vi "CLD 10 Step Sequencer with CSV Front Panel.vi"() -> ()   [LabVIEW 2025]
doc: "CLD 10 Exercise"
uses:
  CLD 10 CSV file enum.ctl
panel:
  out "Elapsed Time (s)":string
  in  "Auto Reset":bool=TRUE
  in  "Reset Button":bool
  in  "Stop VI":bool
  in  "Time Target (s)":dbl
  out "Current Step Time":dbl
  out "Step 1":bool
  out "Step 2":bool
  out "Step 3":bool
  out "Time Has Elapsed":bool
  out "error out":errorcluster
  in  "error in (no error)":errorcluster
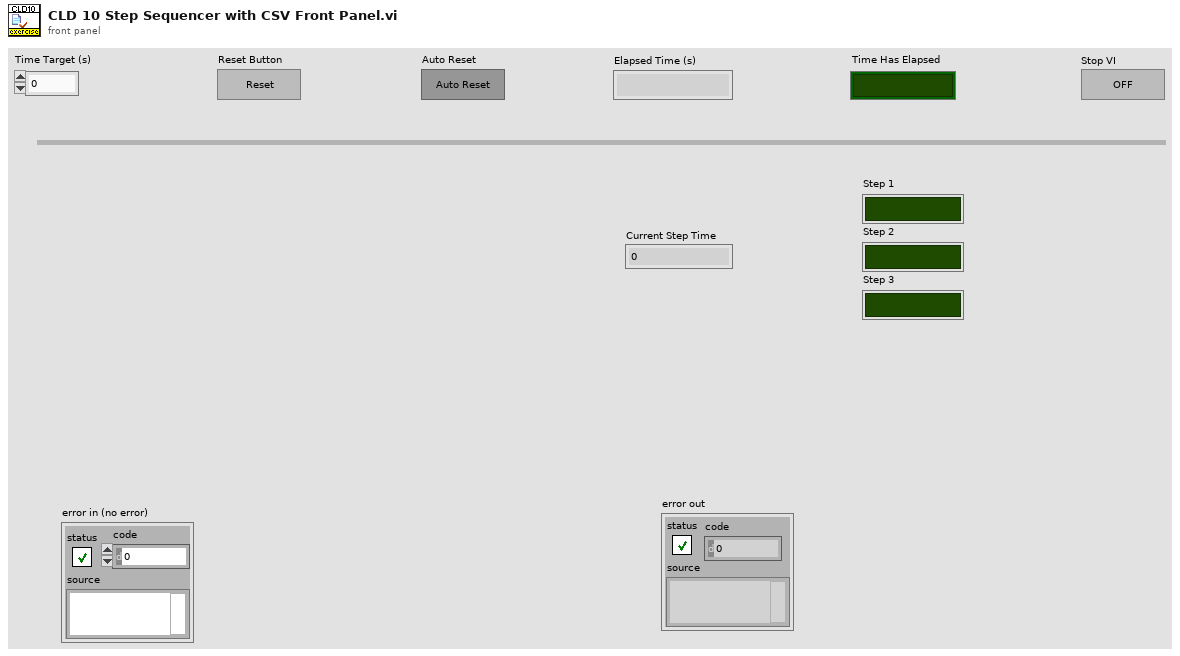
[diagram p1: front panel]
types:
  T1 = typedef "CLD 10 CSV file enum.ctl" = enum16{"Read CSV", "Write CSV"}
  T2 = typedef "CLD 10 CSV file data structure.ctl" = cluster{"Step Time Target":i32, "Step 1":bool, "Step 2":bool, "Step 3":bool}
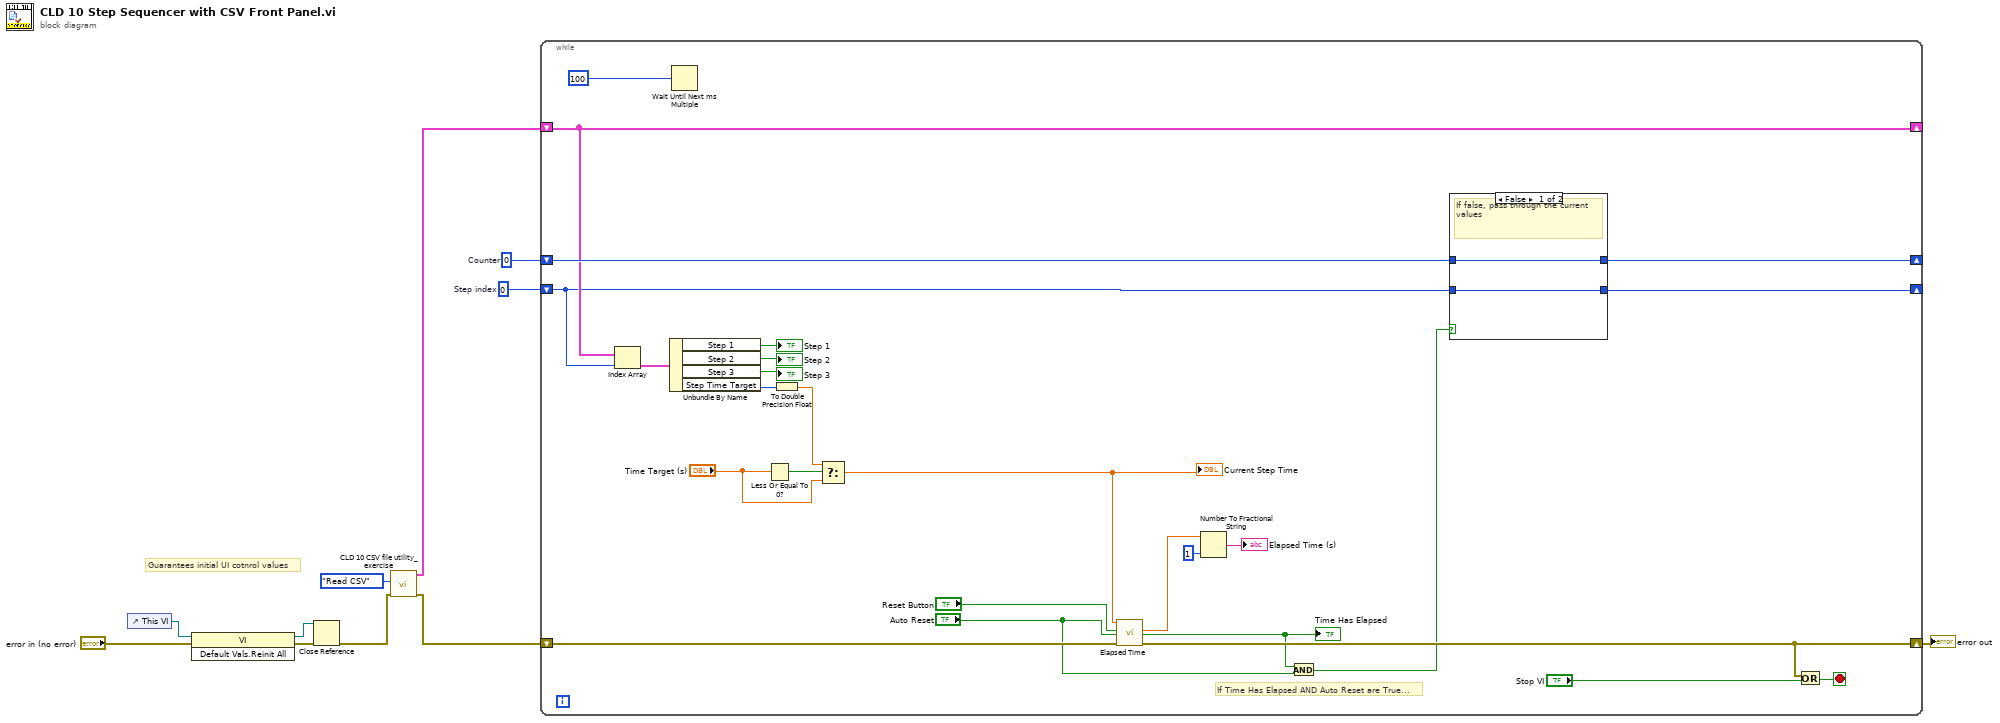
[diagram p0: block diagram]
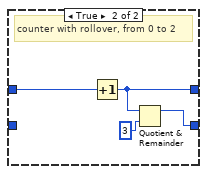
[diagram p2: hidden frame]
diagram:
  w8 = 0  # Step index
  w9 = 0  # Counter
  # "Guarantees initial UI cotnrol values"
  n1 = control-ref of="This VI"() -> (w6:refnum<vi>)
  n2 = invoke class="VI" method="Default Vals.Reinit All"(reference=w6, error in="error in (no error)") -> (reference out=w5:refnum<vi>, error out=w7:errorcluster)  [unwired: 1 in, 1 out]
  n3 = Close Reference(reference=w5, error in (no error)=w7) -> (error out=w2:errorcluster)
  n4 = call "CLD 10 CSV file utility_exercise.vi"("Error In"=w2, "CLD 10 file Enum"=CLD_10_CSV_file_enum."Read CSV") -> ("Error Out"=w1:errorcluster, "[Data Out]"=w3:T2[])  [unwired: 8 in]
  n5 = while {
    shift-right: [w31] -> w10
    shift-left: w1 -> [w37]
    shift-right: [w28] -> _
    shift-left: w9 -> [w29]
    shift-right: [w24] -> _
    shift-left: w8 -> [w21]
    shift-right: [w22] -> _
    shift-left: w3 -> [w22]
    stop <- w32 stop-if-true
    # "If Time Has Elapsed AND Auto Reset are True..."
    n6 = Index Array(array=w22, index=w21) -> (element=w20:T2)
    n7 = Unbundle By Name(w20) -> ("Step 1"=→"Step 1":bool, "Step 2"=→"Step 2":bool, "Step 3"=→"Step 3":bool, "Step Time Target"=w18:i32)
    n8 = Wait Until Next ms Multiple(millisecond multiple=u32 100) -> ()  [unwired: 1 out]
    n9 = Less Or Equal To 0?(x="Time Target (s)") -> (x <= 0?=w19:bool)
    n10 = To Double Precision Float(number=w18) -> (double precision float=w17:dbl)
    n11 = Select(t=w17, s=w19, f="Time Target (s)") -> (s? t:f=w15:dbl)
    "Current Step Time" <- w15
    n12 = call "Elapsed Time"("Time Target (s)"=w15, "Reset"="Reset Button", "Auto Reset"="Auto Reset", "error in (no error)"=w37) -> ("Elapsed Time (s)"=w35:dbl, "Time has Elapsed"=w27:bool, "error out"=w31:errorcluster)  [unwired: 8 in, 5 out]
    "Time Has Elapsed" <- w27
    n13 = Number To Fractional String(number=w35, precision (6)=i16 1) -> (F-format string=→"Elapsed Time (s)":string)  [unwired: 2 in]
    n14 = And(x=w27, y="Auto Reset") -> (x .and. y?=w26:bool)
    n15 = case shown="False" w26 {
      tunnel: [w38 w42] -> w24
      tunnel: w29 -> [w39 w41]
      tunnel: [w39 w40] -> w28
      tunnel: w21 -> [w38 _]
      frame False {
        # "If false, pass through the current values"
      }
      frame True {
        # "counter with rollover, from 0 to 2"
        n16 = Increment(x=w41) -> (x+1=w40:i32)
        n17 = Quotient & Remainder(x=w40, y=3) -> (x-y*floor(x/y)=w42:i32)  [unwired: 1 out]
      }
    }
    n18 = Or(x=w31, y="Stop VI") -> (x .or. y?=w32:bool)
  }
  "error out" <- w10
